vi "Example Simple.vi"() -> ()   [LabVIEW 2010]
uses:
  C:/tf/play/labview/Tinkerforge.dll
  Tinkerforge.dll
panel:
  out "timestamp (ms)":i64
  out "weekday":u8
  out "centisecond":u8
  out "second":u8
  out "minute":u8
  out "hour":u8
  out "day":u8
  out "month":u8
  out "year":i32
  in  "uid":string="XYZ"
  in  "port":i32=4223
  in  "host":string="localhost"
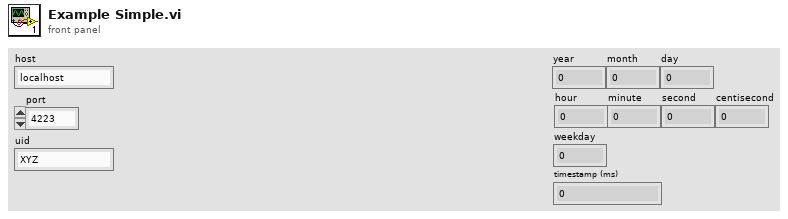
[diagram p1: front panel]
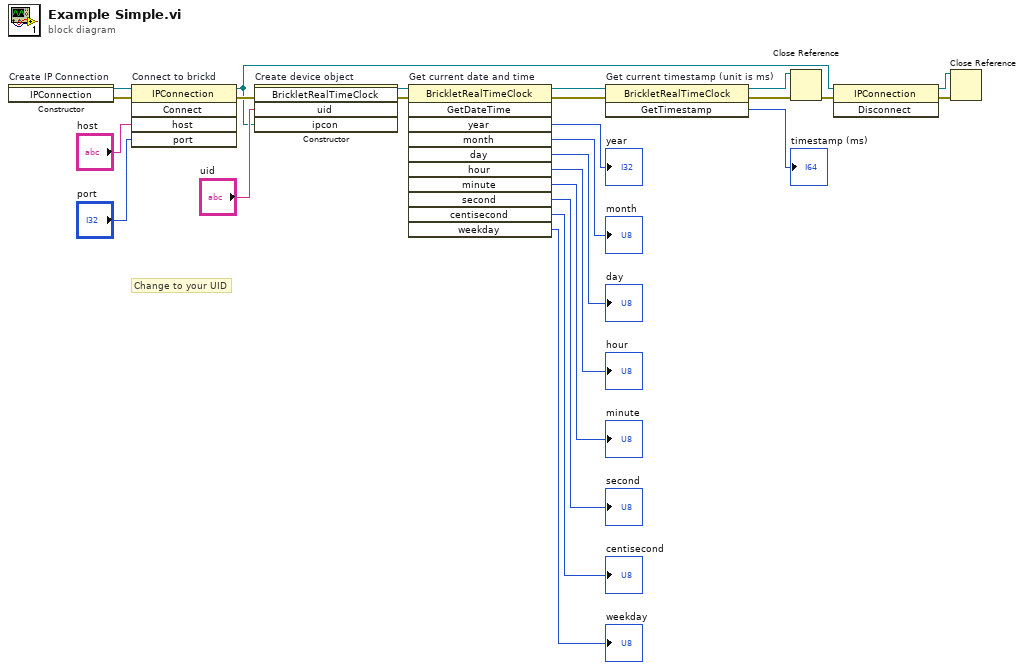
[diagram p0: block diagram]
diagram:
  # "Change to your UID"
  n1 = constructor on="Create IP Connection" class="IPConnection"() -> (reference out=w25:refnum<k24>, error out=w14:errorcluster)  [unwired: 3 in, 1 out]
  n2 = invoke on="Connect to brickd" class="IPConnection" method="Connect"(reference=w25, error in=w14, "host"="host", "port"="port") -> (reference out=w16:refnum<k24>, error out=w21:errorcluster)  [unwired: 1 in, 3 out]
  n3 = constructor on="Create device object" class="BrickletRealTimeClock"(error in=w21, "uid"="uid", "ipcon"=w16) -> (reference out=w19:refnum<k24>, error out=w20:errorcluster)  [unwired: 2 in, 3 out]
  n4 = invoke on="Get current date and time" class="BrickletRealTimeClock" method="GetDateTime"(reference=w19, error in=w20) -> (reference out=w3:refnum<k24>, error out=w4:errorcluster, "year"=→"year":i32, "month"=→"month":u8, "day"=→"day":u8, "hour"=→"hour":u8, "minute"=→"minute":u8, "second"=→"second":u8, "centisecond"=→"centisecond":u8, "weekday"=→"weekday":u8)  [unwired: 9 in, 1 out]
  n5 = invoke on="Get current timestamp (unit is ms)" class="BrickletRealTimeClock" method="GetTimestamp"(reference=w3, error in=w4) -> (reference out=w2:refnum<k24>, error out=w1:errorcluster, "GetTimestamp"=→"timestamp (ms)":i64)  [unwired: 1 in]
  n6 = Close Reference(reference=w2, error in (no error)=w1) -> (error out=w18:errorcluster)
  n7 = invoke class="IPConnection" method="Disconnect"(reference=w16, error in=w18) -> (reference out=w15:refnum<k24>, error out=w17:errorcluster)  [unwired: 1 in, 1 out]
  n8 = Close Reference(reference=w15, error in (no error)=w17) -> ()  [unwired: 1 out]
